vi "Calculate_Compton_Edge.vi"(10 "Spectrum_Array":u16[][](array[numeric]), 11 "Lower Cut-Off":dbl=50.0) -> (3 "Waveform Graph":dbl[][](graph))   [LabVIEW 2019]
uses:
  <vilib>/Analysis/NI_AALPro.lvlib
panel:
  in  "method":u16(ring) items=["2nd Order Central", "4th Order Central", "Forward", "Backward"]
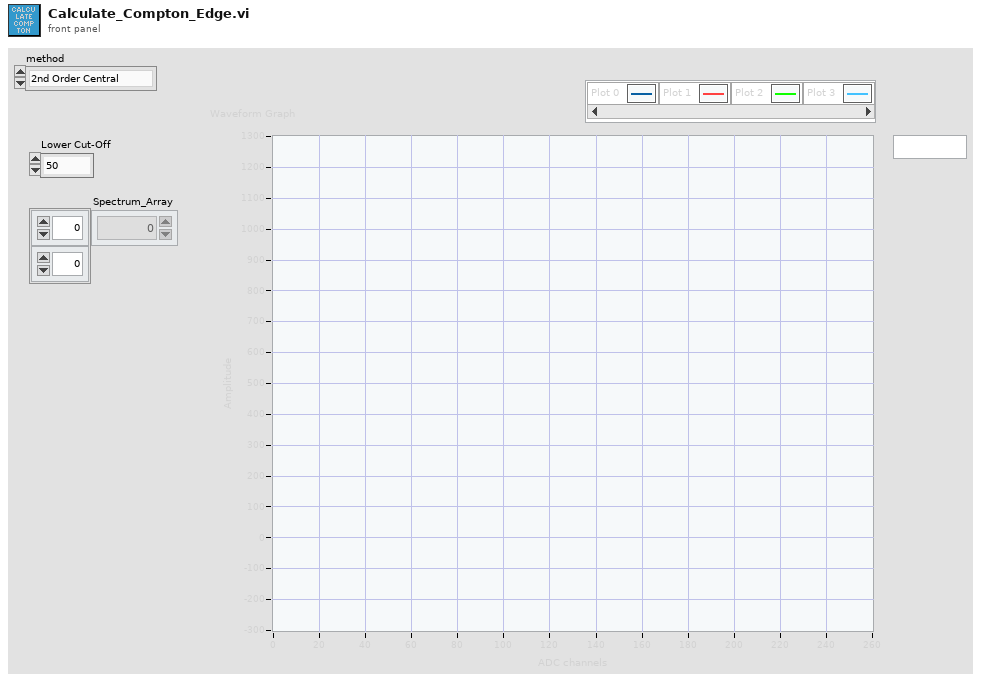
[diagram p1: front panel]
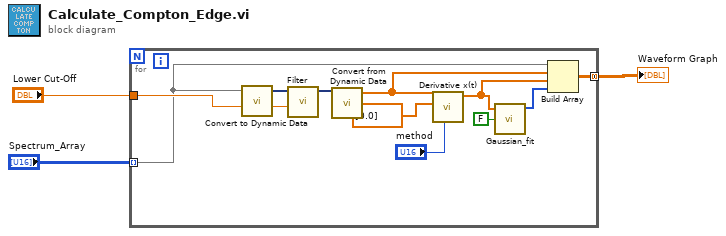
[diagram p0: block diagram]
diagram:
  n1 = for {
    tunnel: "Spectrum_Array" -> [w4] mode=indexing
    tunnel: [w9] -> w2 mode=concatenating
    tunnel: "Lower Cut-Off" -> [w13]
    n2 = call "Convert to Dynamic Data"("Array"=w4) -> ("Dynamic Data Type"=w12:dynamicdata)  [unwired: 3 in]
    n3 = call "Filter"("Lower Cut-Off"=w13, "Signal"=w12) -> ("Filtered Signal"=w11:dynamicdata)  [unwired: 8 in, 1 out]
    n4 = call "Convert from Dynamic Data"("Dynamic Data Type"=w11) -> ("Array"=w10:dbl[])  [unwired: 3 in]
    n5 = call <vilib>:"Derivative x(t).vi"("method"="method", "Initial Condition"=dbl[] [0.0], "X"=w10) -> ("dX/dt"=w7:dbl[])  [unwired: 7 in, 1 out]
    n6 = call "Gaussian_fit.vi"("Input waveform"=w7, "s"=FALSE) -> ("Gaussian fit"=w5:i32[])  [unwired: 4 in, 1 out]
    n7 = Build Array(w4, w10, w7, w5) -> (w9:dbl[][])
  }
  "Waveform Graph" <- w2
